vi "Temperature (c-ºC)(el).vi"(4 "Temperatures in counts":u16) -> (1 "Temperatures in ºC":sgl format="%#.1g ºC")   [LabVIEW 2015, in "VIPM2.lvlib"]
doc: "Chip Temperature conversion from ADC counts to ºC."
uses:
  VIPM2.lvlib
panel:
  # "Conversion Chip Temperatures in counts to ºC"
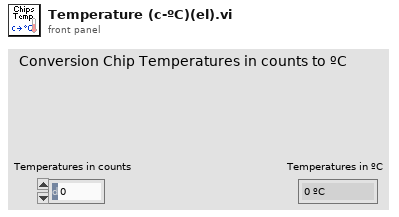
[diagram p1: front panel]
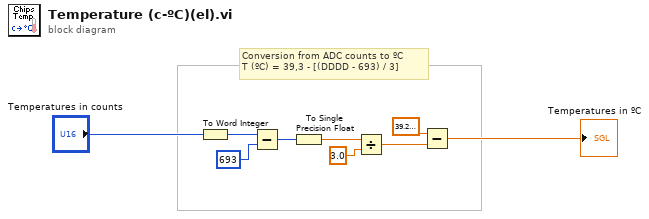
[diagram p0: block diagram]
diagram:
  # "Conversion from ADC counts to ºC\nT (ºC) = 39,3 - [(DDDD - 693) / 3]"
  n1 = To Word Integer(number="Temperatures in counts") -> (16bit integer=w1:i16)
  n2 = Subtract(x=w1, y=i16 693) -> (x-y=w6:i16)
  n3 = To Single Precision Float(number=w6) -> (single precision float=w5:sgl)
  n4 = Divide(x=w5, y=sgl 3.0) -> (x/y=w3:sgl)
  n5 = Subtract(x=sgl 39.3, y=w3) -> (x-y=→"Temperatures in ºC":sgl)
